vi "Seven Segment Counter.vi"() -> ()   [LabVIEW 2025]
panel:
  out "String":string="Seven Segment Display"
  out "Boolean 7":bool
  out "Boolean 6":bool
  out "Boolean 5":bool
  out "Boolean 4":bool
  out "Boolean 3":bool
  out "Boolean 2":bool
  out "Boolean":bool
  in  "Numeric":i32
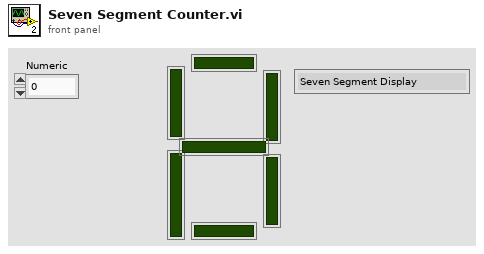
[diagram p1: front panel]
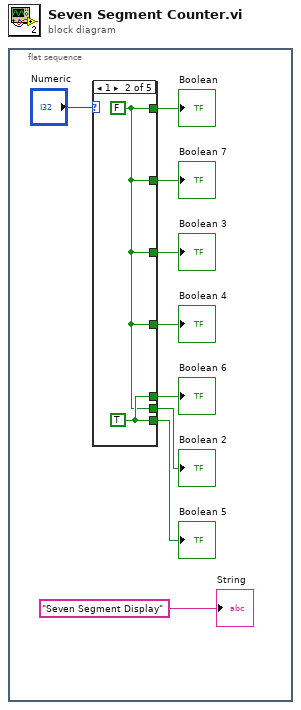
[diagram p0: block diagram]
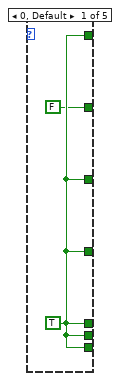
[diagram p2: hidden frame]
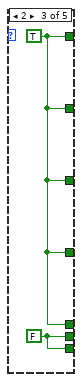
[diagram p3: hidden frame]
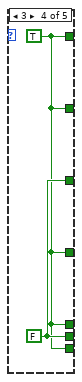
[diagram p4: hidden frame]
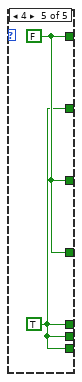
[diagram p5: hidden frame]
diagram:
  n1 = flat-sequence {
    frame #0 {
      n2 = case shown="1" "Numeric" {
        tunnel: [w11 w12 w14 w16 w19] -> w8
        tunnel: [w11 w12 w15 w17 w18] -> w7
        tunnel: [w11 w12 w14 w17 w19] -> w6
        tunnel: [w11 w12 w14 w16 w19] -> w5
        tunnel: [w11 w13 w15 w16 w18] -> w4
        tunnel: [w11 w13 w14 w16 w18] -> w3
        tunnel: [FALSE w12 w14 w16 w18] -> w2
        frame 0, Default {
          w11 = TRUE
        }
        frame 1 {
          w12 = FALSE
          w13 = TRUE
        }
        frame 2 {
          w15 = FALSE
          w14 = TRUE
        }
        frame 3 {
          w17 = FALSE
          w16 = TRUE
        }
        frame 4 {
          w19 = FALSE
          w18 = TRUE
        }
      }
      "Boolean" <- w8
      "Boolean 2" <- w7
      "Boolean 3" <- w6
      "Boolean 5" <- w4
      "Boolean 6" <- w3
      "Boolean 7" <- w2
      "Boolean 4" <- w5
      "String" <- "Seven Segment Display"
    }
  }
